vi "Automated-Hydroponics-1.vi"() -> ()   [LabVIEW 2020]
uses:
  D:/Btech/Semesters/5_sem/Lab_SIP/laTEX/Week_10/Control 1.ctl
panel:
  out "Plants 3":picture
  out "?":bool
  out "?":bool
  out "?":bool
  out "?":bool
  out "Motor on 2":picture
  out "?":bool
  out "?":bool
  out "?":bool
  out "?":bool
  in  "stop":bool
  out "?":bool
  out "Plants 2":picture
  out "Plants":picture
  out "?":bool
  out "?":bool
  out "?":bool
  out "?":bool
  out "?":T1
  out "?":bool
  out "Tank":dbl(slide) scale=0.0..10.0
  out "Motor on":picture
  out "Reservoir":dbl(slide) scale=0.0..20.0
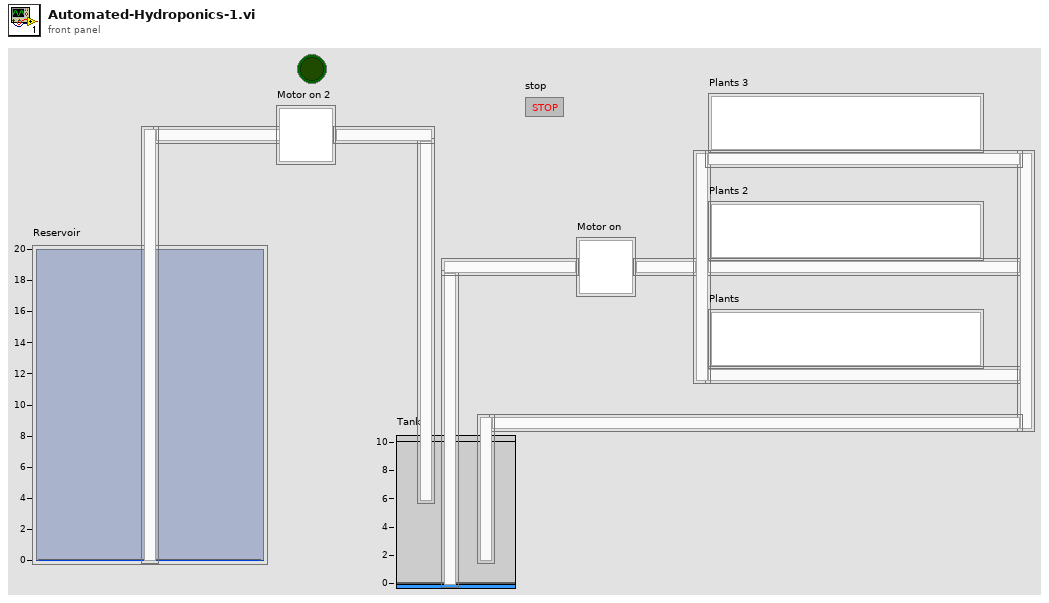
[diagram p1: front panel]
types:
  T1 = typedef "Control 1.ctl" = bool
  T2 = typedef "imagedata.ctl" = cluster{"image type":i32, "image depth":i32, "image":u8[], "mask":u8[], "colors":u32[], "Rectangle":cluster{"left":i16, "top":i16, "right":i16, "bottom":i16}}
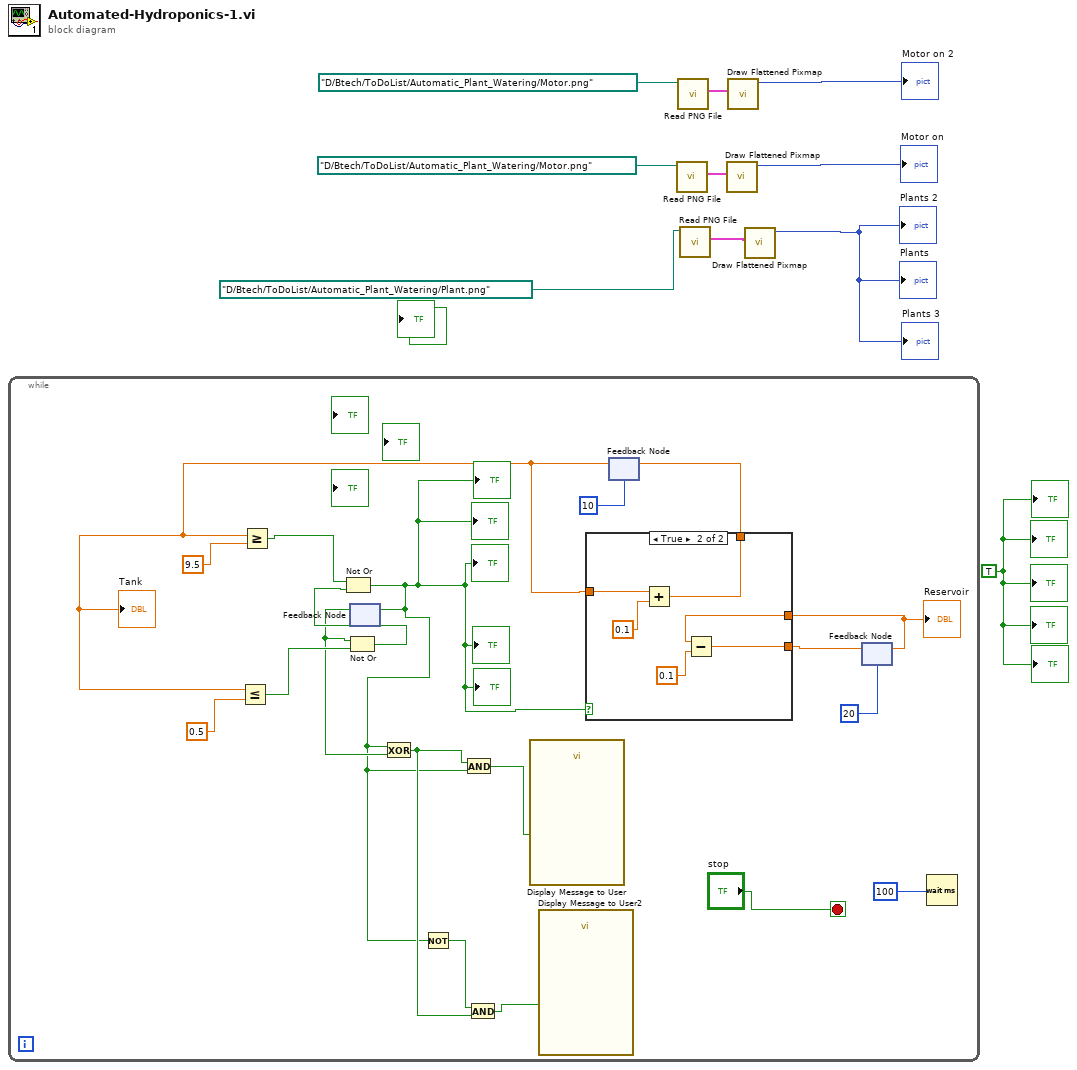
[diagram p0: block diagram]
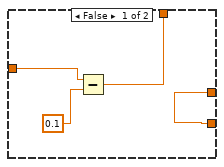
[diagram p2: hidden frame]
diagram:
  w2 = TRUE
  n1 = while {
    stop <- "stop" stop-if-true
    n2 = feedback #1() -> (w17:bool)  [unwired: 1 in]
    n3 = feedback #2(10) -> (w23:dbl)
    "Tank" <- w23
    n4 = Less Or Equal?(x=w23, y=0.5) -> (x <= y?=w26:bool)
    n5 = Greater Or Equal?(x=w23, y=9.5) -> (x >= y?=w25:bool)
    n6 = Not Or(1:w26, 2:w17) -> (0:w27:bool)
    n7 = Not Or(1:w27, 2:w25) -> (0:w12:bool)
    "?" <- w12
    "?" <- w12
    "?" <- w12
    "?" <- w12
    "?" <- w12
    n8 = feedback-in #1(w12) -> ()
    n9 = Exclusive Or(1:w17, 2:w12) -> (0:w13:bool)
    n10 = Not(x=w12) -> (.not. x?=w14:bool)
    n11 = And(x=w13, y=w12) -> (x .and. y?=w16:bool)
    n12 = And(x=w14, y=w13) -> (x .and. y?=w15:bool)
    n13 = call "Display Message to User"("Enable"=w16) -> ()  [unwired: 9 in, 2 out]
    n14 = call "Display Message to User2"("Enable"=w15) -> ()  [unwired: 9 in, 2 out]
    n15 = feedback #3(20) -> (w19:dbl)
    "Reservoir" <- w19
    n16 = case shown="True" w12 {
      tunnel: w23 -> [w33 w39]
      tunnel: [w31 w37] -> w24
      tunnel: w19 -> [w30 w36]
      tunnel: [w30 w34] -> w20
      frame False {
        n17 = Subtract(x=w33, y=0.1) -> (x-y=w31:dbl)
      }
      frame True {
        n18 = Add(x=w39, y=0.1) -> (x+y=w37:dbl)
        n19 = Subtract(x=w36, y=0.1) -> (x-y=w34:dbl)
      }
    }
    n20 = feedback-in #2(w24) -> ()
    n21 = feedback-in #3(w20) -> ()
    n22 = Wait (ms)(milliseconds to wait=100) -> ()  [unwired: 1 out]
  }
  n23 = call <vilib>:"Read PNG File.vi"("path to PNG file"=path "D:/Btech/ToDoList/Automatic_Plant_Watering/Motor.png") -> ("image data"=w9:T2)  [unwired: 8 in, 2 out]
  n24 = call <vilib>:"Read PNG File.vi"("path to PNG file"=path "D:/Btech/ToDoList/Automatic_Plant_Watering/Motor.png") -> ("image data"=w4:T2)  [unwired: 8 in, 2 out]
  n25 = call <vilib>:"Read PNG File.vi"("path to PNG file"=path "D:/Btech/ToDoList/Automatic_Plant_Watering/Plant.png") -> ("image data"=w7:T2)  [unwired: 8 in, 2 out]
  n26 = call <vilib>:"Draw Flattened Pixmap.vi"("image data"=w9) -> ("new picture"=→"Motor on":picture)  [unwired: 8 in]
  n27 = call <vilib>:"Draw Flattened Pixmap.vi"("image data"=w4) -> ("new picture"=→"Motor on 2":picture)  [unwired: 8 in]
  n28 = call <vilib>:"Draw Flattened Pixmap.vi"("image data"=w7) -> ("new picture"=→"Plants" →"Plants 2" →"Plants 3":picture)  [unwired: 8 in]
  "?" <- w2
  "?" <- w2
  "?" <- w2
  "?" <- w2
  "?" <- w2
